vi "Accordeur Face Avant_BELKACEMI_NDIAYE.vi"() -> ()   [LabVIEW 2024]
uses:
  <vilib>/measure/matone.llb/Extract Single Tone Information N Chan.vi
  <vilib>/measure/NI_MABase.lvlib
  <vilib>/measure/NI_MAPro.lvlib
panel:
  in  "Note d'accord":dbl(ring) items=["MI grave"=330.0, "LA"=440.0, "RE"=587.0, "SOL"=784.0, "SI"=987.0, "MI aigu"=1318.5]
  out "LED ROUGE":bool
  out "LED ORANGE":bool
  out "LED VERTE":bool
  out "Chaîne":string
  out "Amplitude battement":dbl(knob) scale=0.0..10.0
  out "Signal de battement":dynamicdata(graph)
  out "Signal Instrument":dynamicdata(graph)
  out "Signal d'accord":waveform(dbl)(graph)
  # "ACCORDEUR DE FREQUENCE"
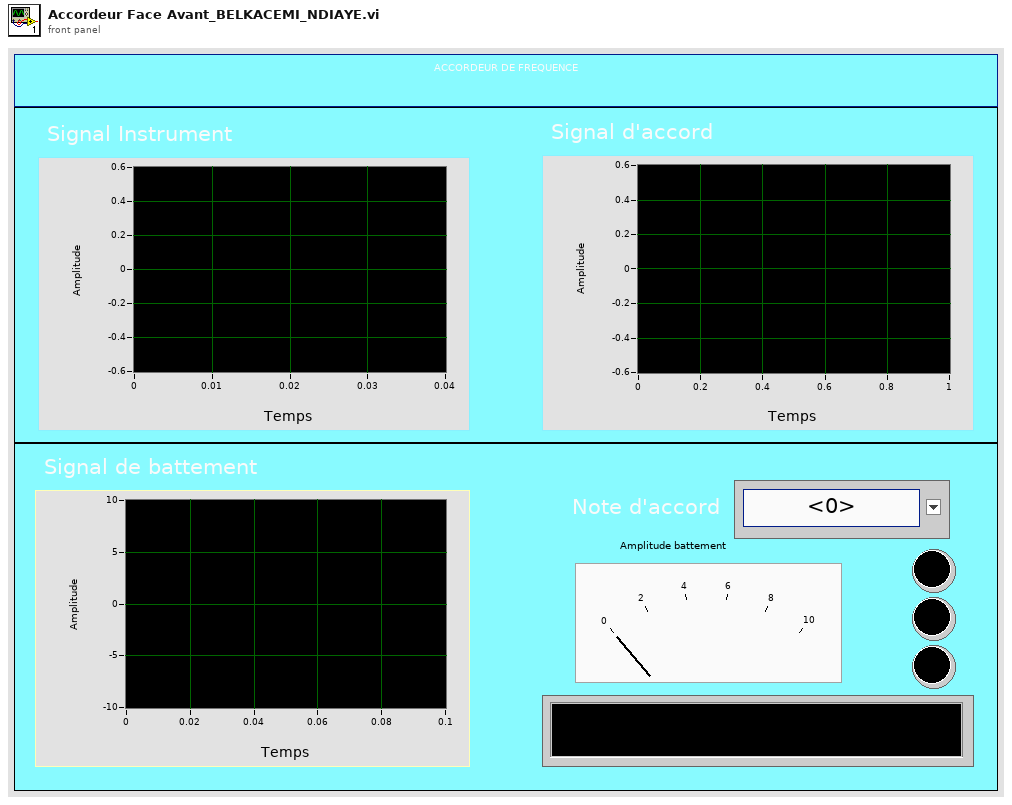
[diagram p1: front panel]
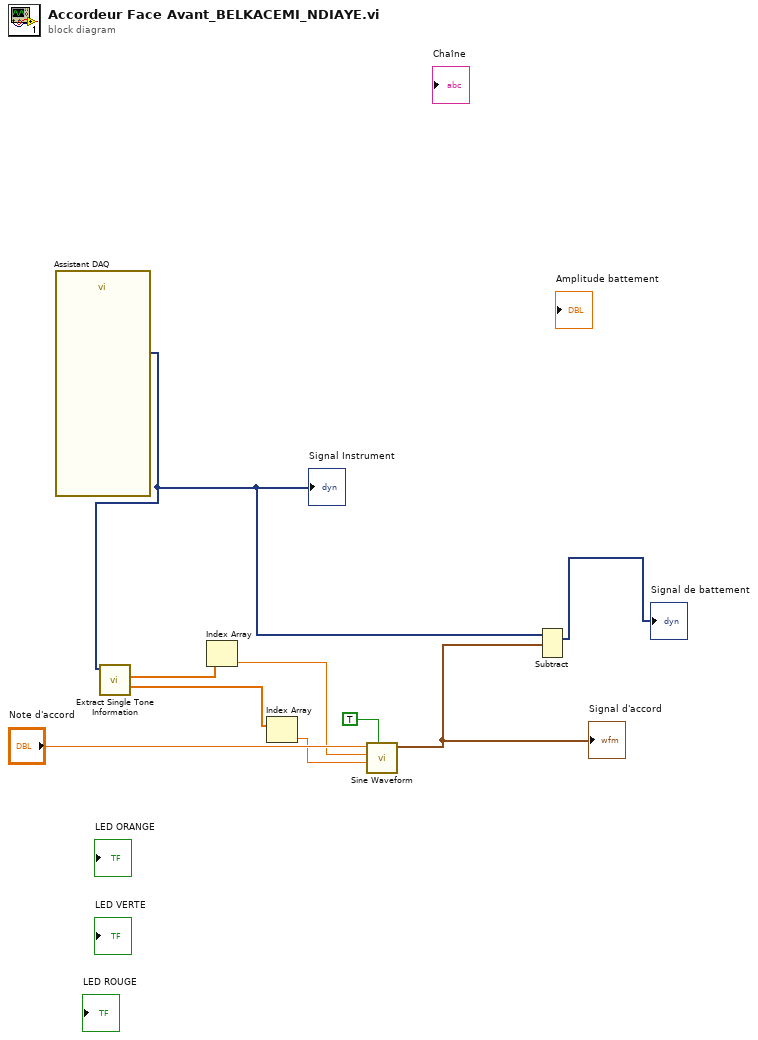
[diagram p0: block diagram]
diagram:
  n1 = call "Assistant DAQ"() -> ("data"=w6:dynamicdata)  [unwired: 17 in, 2 out]
  "Signal Instrument" <- w6
  n2 = call-poly <vilib>:"Extract Single Tone Information.vi"("time signals in"=w6) -> ("detected phases (deg)"=w4:dbl[], "detected amplitudes"=w5:dbl[])  [unwired: 5 in, 4 out]
  n3 = Index Array(array=w5) -> (element=w7:dbl)  [unwired: 1 in]
  n4 = Index Array(array=w4) -> (element=w3:dbl)  [unwired: 1 in]
  n5 = call <vilib>:"Sine Waveform.vi"("reset signal"=TRUE, "phase"=w3, "amplitude"=w7, "frequency"="Note d'accord") -> ("signal out"=w8:waveform(dbl))  [unwired: 6 in, 1 out]
  "Signal d'accord" <- w8
  n6 = Subtract(1:w8, 2:w6) -> (0:→"Signal de battement":dynamicdata)  [unwired: 1 in, 1 out]
